vi "DAT to LV.vi"(6 "header length":i32=11, 8 "error in (no error)":errorcluster, 11 "File Path":path) -> (0 "error out":errorcluster, 2 "Wavenames":string[](array[string]), 3 "Data":dbl[][](array[numeric]), 4 "Comments":string)   [LabVIEW 2016, in "LVtoITX.lvclass"]
uses:
  LVtoITX.lvclass
  <vilib>/Utility/file.llb/Read Delimited Spreadsheet (string).vi
panel:
  out "all rows":string[][](array[string])
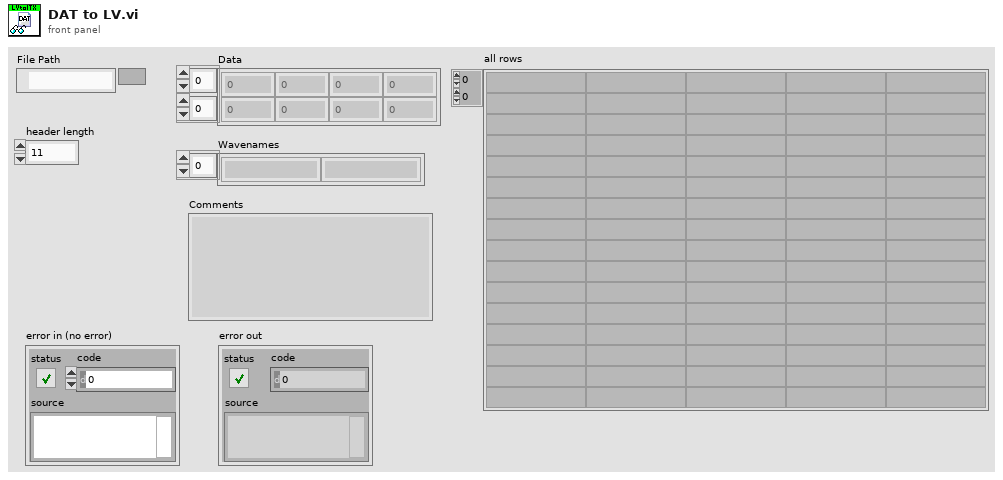
[diagram p1: front panel]
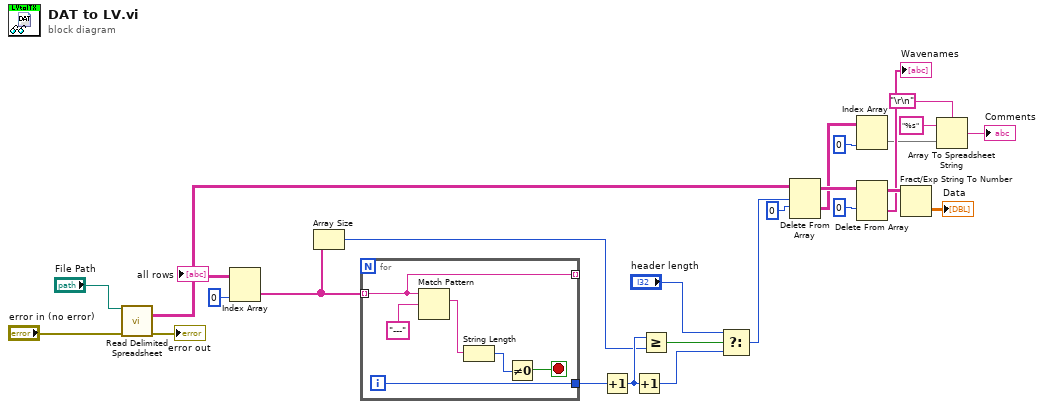
[diagram p0: block diagram]
diagram:
  n1 = call-poly <vilib>:"Read Delimited Spreadsheet.vi"("file path (dialog if empty)"="File Path", "error in (no error)"="error in (no error)") -> ("all rows"=w10:string[][], "error out"=→"error out":errorcluster)  [unwired: 8 in, 4 out]
  "all rows" <- w10
  n2 = Index Array(array=w10, index (col)=0 ("disabled index (col)")) -> (element=w7:string[])  [unwired: 1 in]
  n3 = Array Size(array=w7) -> (size(s)=w4:i32)
  n4 = for {
    tunnel: w7 -> [w26] mode=indexing
    tunnel: [w27] -> w8
    tunnel: [w26] -> _ mode=indexing
    i -> [w27]
    stop <- w29 stop-if-true
    n5 = Match Pattern(string=w26, regular expression="---") -> (match substring=w30:string)  [unwired: 4 out]
    n6 = String Length(string=w30) -> (length=w28:i32)
    n7 = Not Equal To 0?(x=w28) -> (x != 0?=w29:bool)
  }
  n8 = Increment(x=w8) -> (x+1=w6:i32)
  n9 = Increment(x=w6) -> (x+1=w3:i32)
  n10 = Greater Or Equal?(x=w6, y=w4) -> (x >= y?=w5:bool)
  n11 = Select(t="header length", s=w5, f=w3) -> (s? t:f=w1:i32)
  n12 = Delete From Array(array=w10, length=w1, index (row)=0) -> (deleted portion=w14:string[][], array with subset deleted=w21:string[][])  [unwired: 1 in]
  n13 = Index Array(array=w14, index (col)=0 ("disabled index (col)")) -> (element=w13:string[])  [unwired: 1 in]
  n14 = Delete From Array(array=w21, index (row)=0) -> (deleted portion=→"Wavenames":string[], array with subset deleted=w23:string[][])  [unwired: 2 in]
  n15 = Fract/Exp String To Number(string=w23) -> (number=→"Data":dbl[][])  [unwired: 3 in, 1 out]
  n16 = Array To Spreadsheet String(delimiter (Tab)="\r\n", array=w13, 3:"%s" ("format string")) -> (spreadsheet string=→"Comments":string)
